vi "test_trigger_delay.vi"() -> ()   [LabVIEW 2018]
panel:
  out "Waveform Graph":i16[](graph)
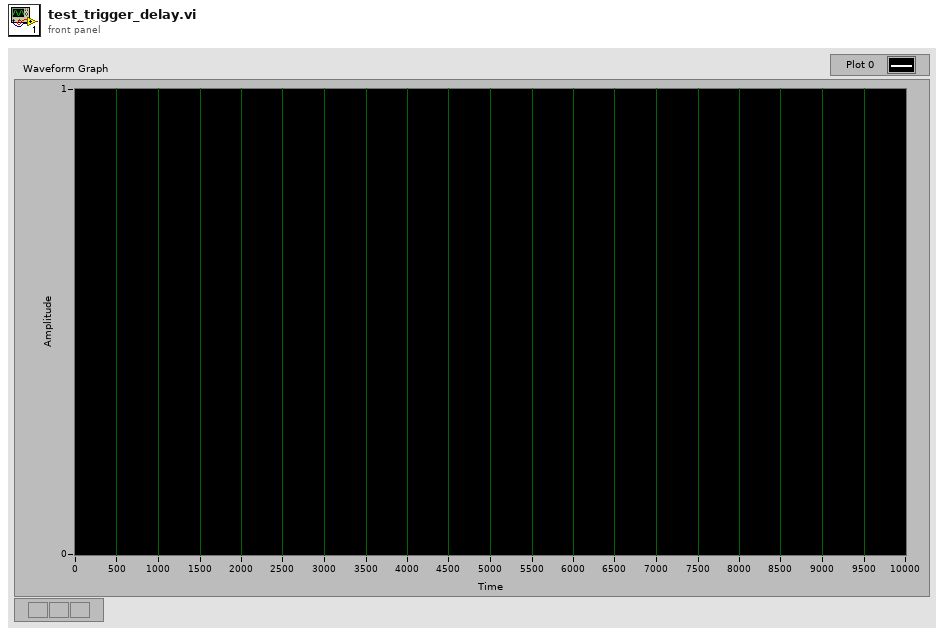
[diagram p1: front panel]
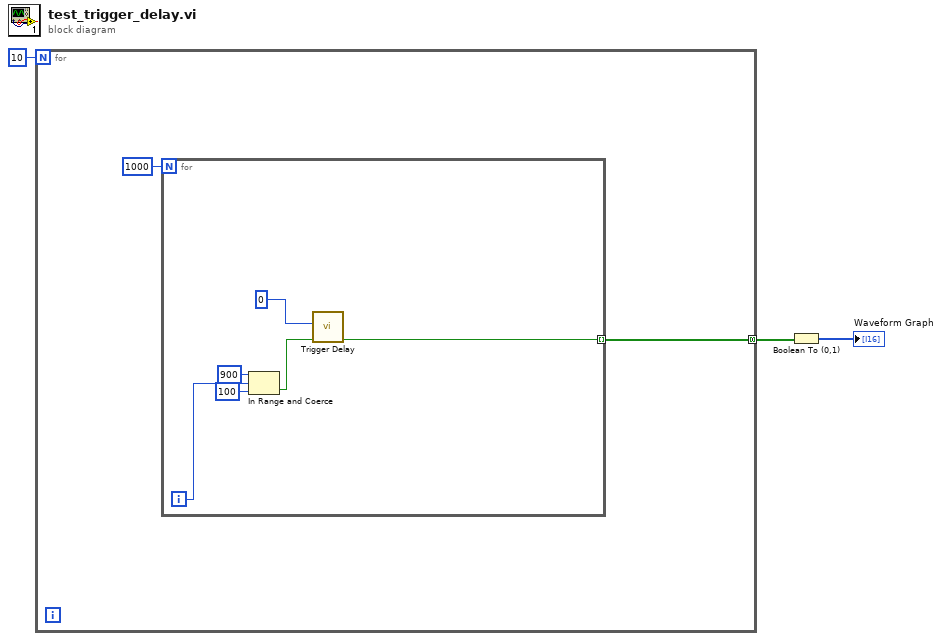
[diagram p0: block diagram]
diagram:
  n1 = for {
    N: 10 -> [_]
    tunnel: [w4] -> w2 mode=concatenating
    n2 = for {
      N: 1000 -> [_]
      tunnel: [w11] -> w4 mode=indexing
      i -> [w9]
      n3 = In Range and Coerce(upper limit=900, x=w9, lower limit=100) -> (In Range?=w6:bool)  [unwired: 1 out]
      n4 = call "Trigger Delay.vi"("input valid"=w6, "Count to skip"=u32 0) -> ("output valid"=w11:bool)  [unwired: 9 in]
    }
  }
  n5 = Boolean To (0,1)(Boolean=w2) -> (0, 1=→"Waveform Graph":i16[])
